vi "report-test-results.vi"(8 "error in (no error)":errorcluster, 9 "TestPassed":bool, 11 "Test Name":string) -> (0 "error out":errorcluster)   [LabVIEW 2019]
uses:
  <vilib>/Rock Robotics/Network Tables/NT Write String.vi
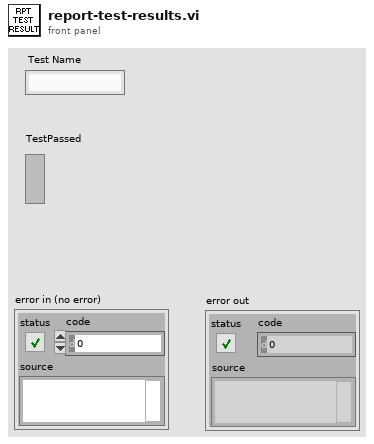
[diagram p1: front panel]
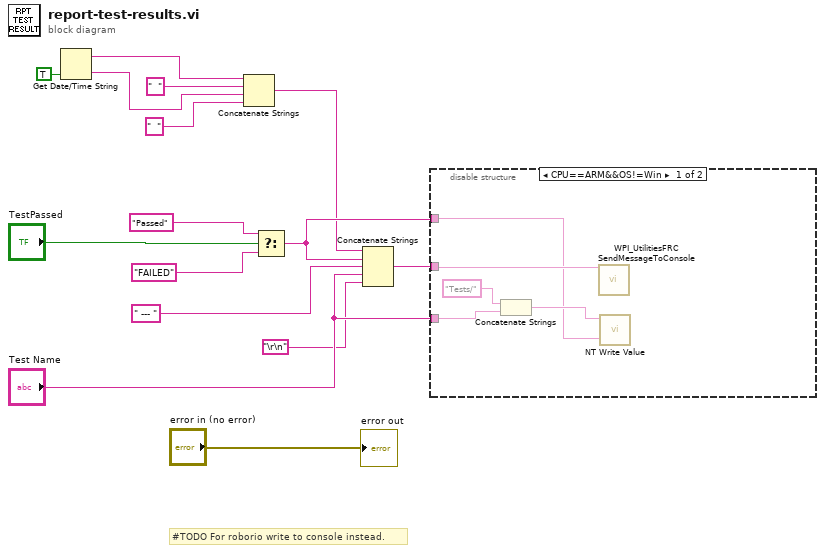
[diagram p0: block diagram]
diagram:
  # "#TODO For roborio write to console instead."
  n1 = Get Date/Time String(want seconds? (F)=TRUE) -> (date string=w5:string, time string=w3:string)  [unwired: 2 in]
  n2 = Concatenate Strings(w5, "  " ("string"), w3, "  " ("string")) -> (w1:string)
  n3 = Select(t="Passed", s="TestPassed", f="FAILED") -> (s? t:f=w9:string)
  n4 = Concatenate Strings(w1, w9, " --- ", "Test Name", "\r\n") -> (w11:string)
  n5 = disable-structure shown="CPU==ARM&&OS!=Win" {
    disable-tunnel: w11 -> [w20 _]
    disable-tunnel: "Test Name" -> [w18 _]
    disable-tunnel: w9 -> [w16 _]
    frame condition #0 {
      n6 = Concatenate Strings("Tests/" ("string"), w18) -> (w17:string)
      n7 = call <vilib>:"WPI_UtilitiesFRC SendMessageToConsole.vi"("Message"=w20) -> ()  [unwired: 14 in, 1 out]
      n8 = call-poly <vilib>:"NT Write Value.vi"("String"=w16, "Name"=w17) -> ()  [unwired: 9 in, 1 out]
    }
    frame condition #1 (active) {
    }
  }
  "error out" <- "error in (no error)"
